vi "Standby Power Data Process.vi"(7 "Loop Index":i32, 8 "Error In":errorcluster, 9 "Standby Power In in":T1, 10 "Total Array Input":string[][](array[string]), 11 "Array DBL":dbl[][](array[numeric])) -> (0 "Error Out":errorcluster, 1 "Standby Power In out":T1, 2 "Plot Data":string[][](array[string]), 4 "Average Data":string[][](array[string]))   [LabVIEW 2018]
uses:
  Type Definitions/Standby Power Main Data.ctl
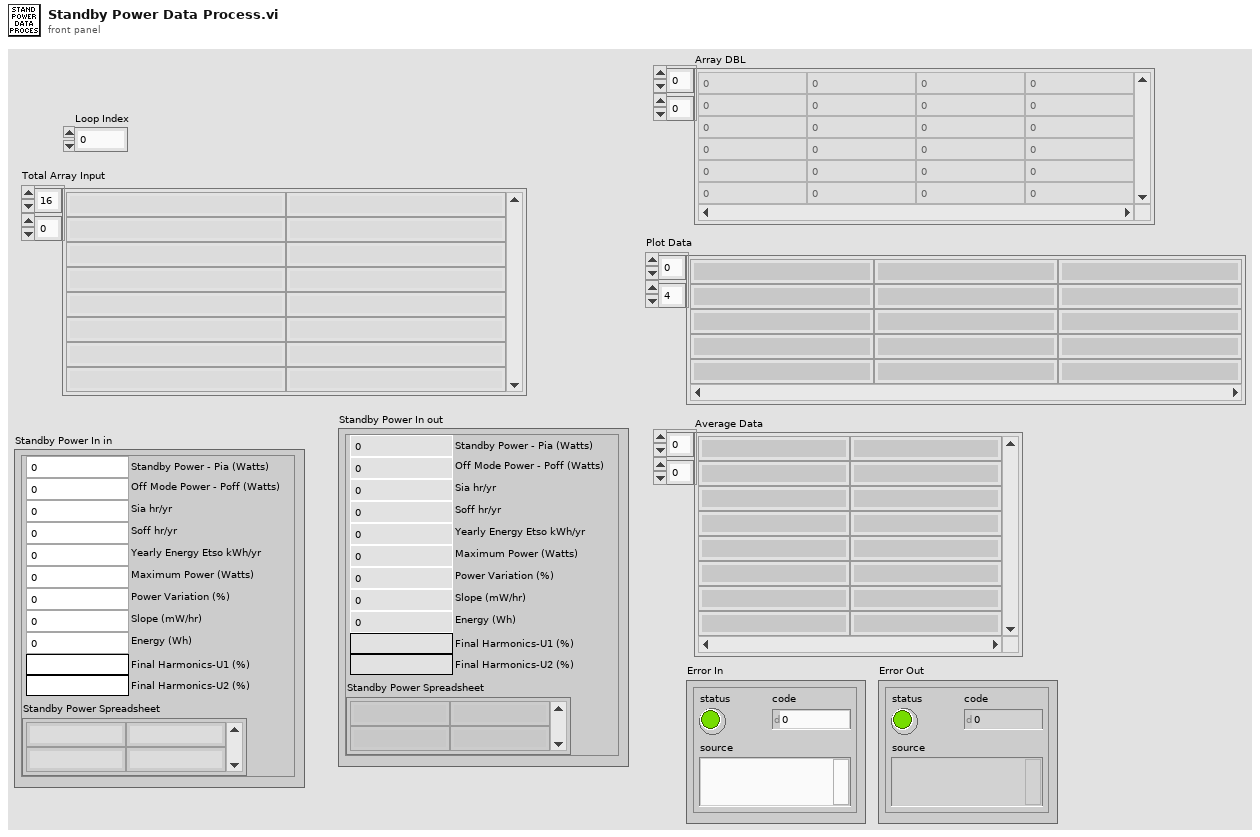
[diagram p1: front panel]
types:
  T1 = typedef "Standby Power Main Data.ctl" = cluster{"Standby Power Spreadsheet":string[][], "Standby Power - Pia (Watts)":dbl, "Off Mode Power - Poff (Watts)":dbl, "Sia hr/yr":dbl, "Soff hr/yr":dbl, "Yearly Energy Etso kWh/yr":dbl, "Maximum Power (Watts)":dbl, "Power Variation (%)":dbl, "Slope (mW/hr)":dbl, "Final Harmonics-U1 (%)":string, "Final Harmonics-U2 (%)":string, "Energy (Wh)":dbl}
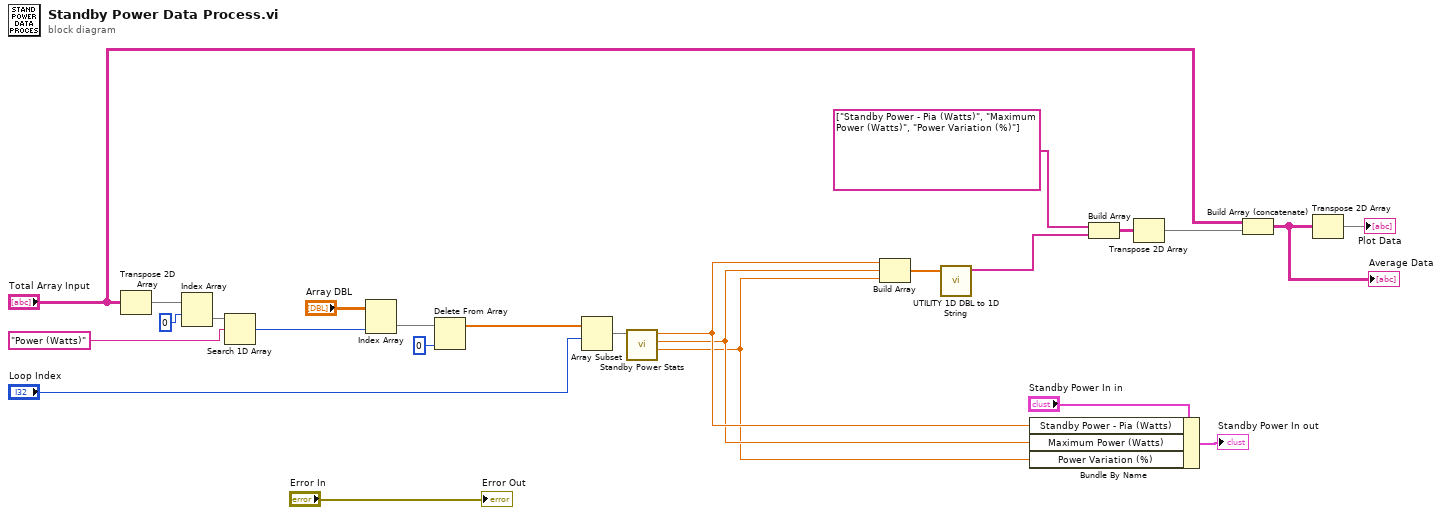
[diagram p0: block diagram]
diagram:
  n1 = Transpose 2D Array(2D array="Total Array Input") -> (transposed array=w7:string[][])
  n2 = Index Array(array=w7, index (row)=0 ("disabled index (col)")) -> (element=w22:string[])  [unwired: 1 in]
  n3 = Search 1D Array(1D array=w22, element="Power (Watts)") -> (index of element=w20:i32)  [unwired: 1 in]
  n4 = Index Array(array="Array DBL", index (col)=w20) -> (element=w17:dbl[])  [unwired: 1 in]
  n5 = Delete From Array(array=w17, index=0) -> (array with subset deleted=w8:dbl[])  [unwired: 1 in, 1 out]
  n6 = Array Subset(array=w8, index="Loop Index") -> (w19:dbl[])  [unwired: 1 in]
  n7 = call "Standby Power Stats.vi"("Full Data Array"=w19) -> ("Power Variation (%)"=w13:dbl, "Maximum Power (Watts)"=w14:dbl, "Standby Power - Pia (Watts)"=w15:dbl)  [unwired: 7 in, 1 out]
  n8 = Build Array(w15, w14, w13) -> (w12:dbl[])
  n9 = call "UTILITY 1D DBL to 1D String.vi"("1D DBL"=w12) -> ("1D String"=w11:string[])  [unwired: 10 in]
  n10 = Bundle By Name(cluster="Standby Power In in", "Standby Power - Pia (Watts)"=w15, "Maximum Power (Watts)"=w14, "Power Variation (%)"=w13) -> (→"Standby Power In out":T1)
  n11 = Build Array(string[] ["Standby Power - Pia (Watts)", "Maximum Power (Watts)", "Power Variation (%)"], w11) -> (w6:string[][])
  n12 = Transpose 2D Array(2D array=w6) -> (transposed array=w5:string[][])
  n13 = Build Array (concatenate)("Total Array Input", w5) -> (w1:string[][])
  "Average Data" <- w1
  n14 = Transpose 2D Array(2D array=w1) -> (transposed array=→"Plot Data":string[][])
  "Error Out" <- "Error In"
